vi "destroyEvents.vi"(8 "error in (no error)":errorcluster, 11 "SnapperEvents in":refnum<class "SnapperEvents.lvclass">) -> (0 "error out":errorcluster, 3 "SnapperEvents out":refnum<class "SnapperEvents.lvclass">)   [LabVIEW 2011, in "Views.lvlib" / "Camera.lvlib" / "SnapperEvents.lvclass"]
uses:
  SnapperEvents.lvclass
  SnapperEvents.lvclass/SnapperEvents.ctl
  Camera.lvlib
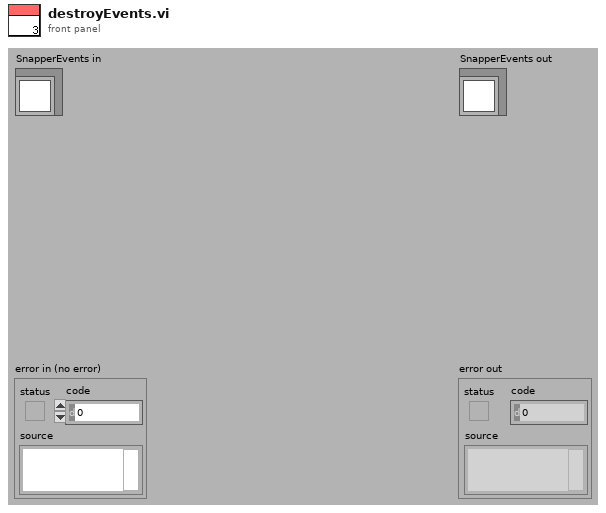
[diagram p1: front panel]
types:
  T1 = cluster{"frontEndEvents":cluster{"snapShotEvent":refnum<user-event>, "stopShooting":refnum<user-event>, "userSnapShot":refnum<user-event>}, "backEndEvents":cluster{"picture":refnum<user-event>}}
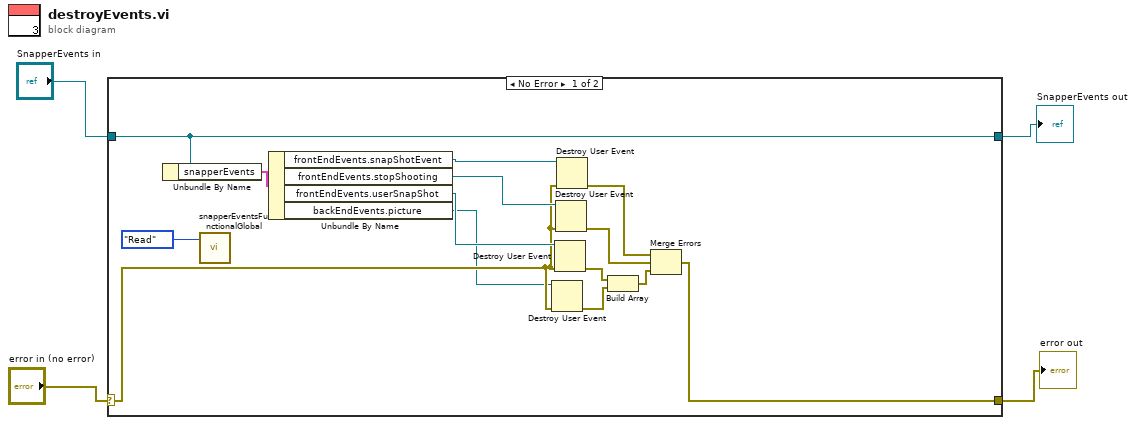
[diagram p0: block diagram]
diagram:
  n1 = case shown="No Error" "error in (no error)" {
    selector: "error in (no error)" -> [w9 w20]
    tunnel: [w17 w20] -> w1
    tunnel: [w11 w19] -> w2
    tunnel: "SnapperEvents in" -> [w11 w19]
    frame No Error {
      n2 = Unbundle By Name(w11) -> ("snapperEvents"=w10:T1)
      n3 = call "snapperEventsFunctionalGlobal.vi"("Action"=enum16{"Write", "Read"}."Read") -> ()  [unwired: 10 in, 1 out]
      n4 = Unbundle By Name(w10) -> ("frontEndEvents.snapShotEvent"=w16:refnum<user-event>, "frontEndEvents.stopShooting"=w15:refnum<user-event>, "frontEndEvents.userSnapShot"=w14:refnum<user-event>, "backEndEvents.picture"=w8:refnum<user-event>)
      n5 = Destroy User Event(user event=w8, error in=w9) -> (error out=w6:errorcluster)
      n6 = Destroy User Event(user event=w14, error in=w9) -> (error out=w7:errorcluster)
      n7 = Destroy User Event(user event=w15, error in=w9) -> (error out=w12:errorcluster)
      n8 = Destroy User Event(user event=w16, error in=w9) -> (error out=w13:errorcluster)
      n9 = Build Array(w7, w6) -> (w5:errorcluster[])
      n10 = Merge Errors(w13, w12, w5) -> (w17:errorcluster)
    }
    frame Error {
    }
  }
  "error out" <- w1
  "SnapperEvents out" <- w2
